vi "Signal Constructor.vi"(8 "error in (no error)":errorcluster, 11 "Signal Settings":T1) -> (0 "error out":errorcluster, 3 "IO Class.lvclass":refnum<class "Signal.lvclass">)   [LabVIEW 2015, in "Signal.lvclass"]
uses:
  Signal.lvclass
  Signal Settings.ctl
  Configuration.ctl
  Digital Indicator/Digital Indicator.lvclass
  Digital Control/Digital Control.lvclass
  Analog Indicator/Analog Indicator.lvclass
  Analog Control/Analog Control.lvclass
  FPGA Addon Input/FPGA Addon Input.lvclass
  FPGA Addon Output/FPGA Addon Output.lvclass
  Wheel Speed Sensor/Wheel Speed Sensor.lvclass
  Signal.lvclass/Signal.ctl
  EST Digital Event/Digital Event.lvclass
  EST Output/EST Output.lvclass
  EST Knock Sensor/Knock Sensor.lvclass
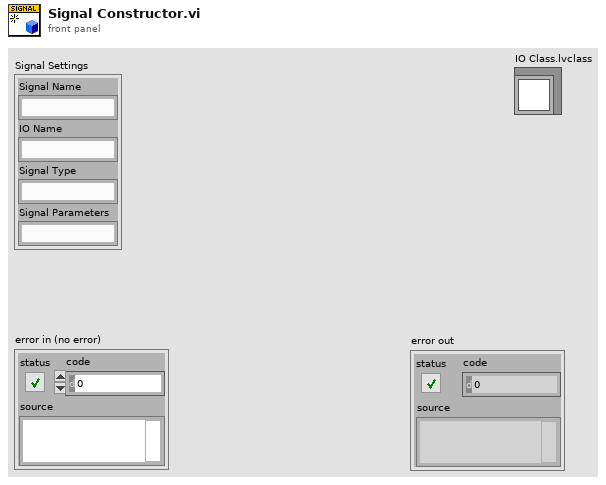
[diagram p1: front panel]
types:
  T1 = typedef "Signal.lvclass/Signal Settings.ctl" = cluster{"Signal Name":string, "IO Name":string, "Signal Type":string, "Signal Parameters":string}
  T2 = typedef "Signal.lvclass/Configuration.ctl" = cluster{"Classification":string, "Direction":string, "Type":string}
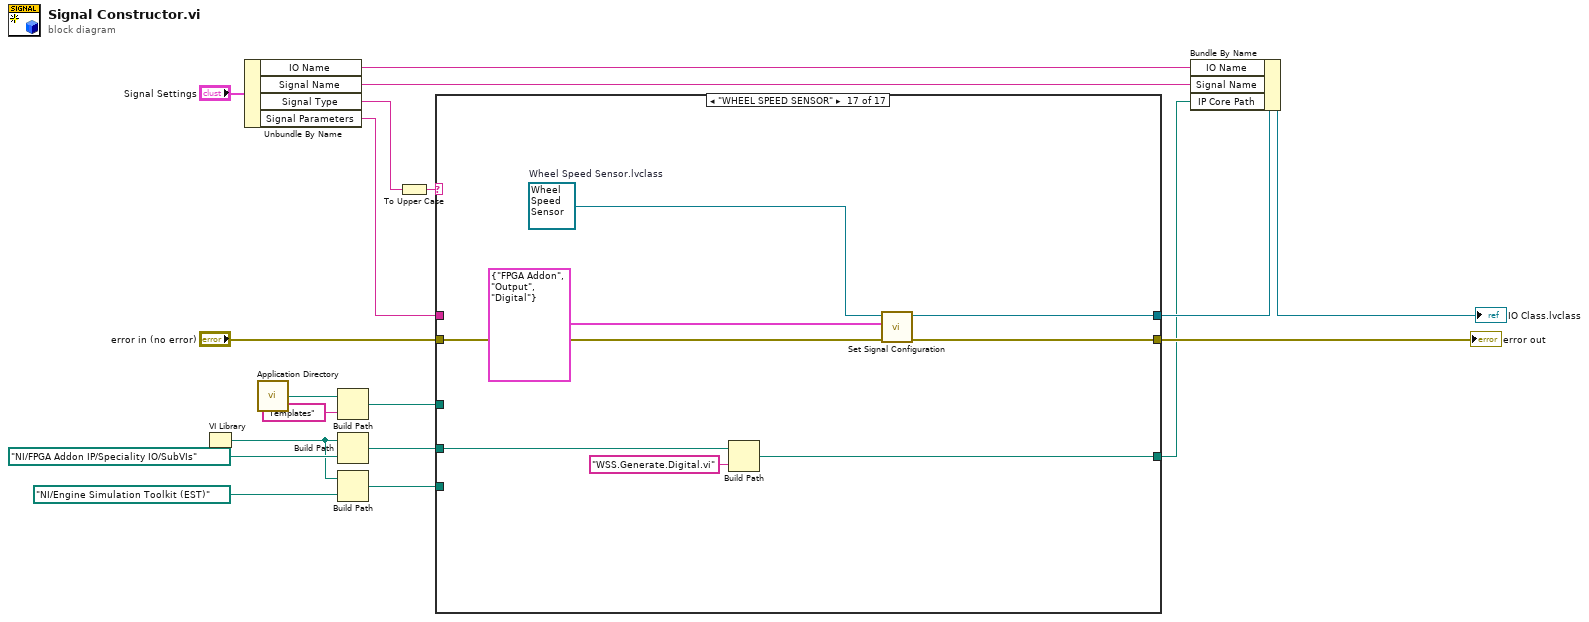
[diagram p0: block diagram]
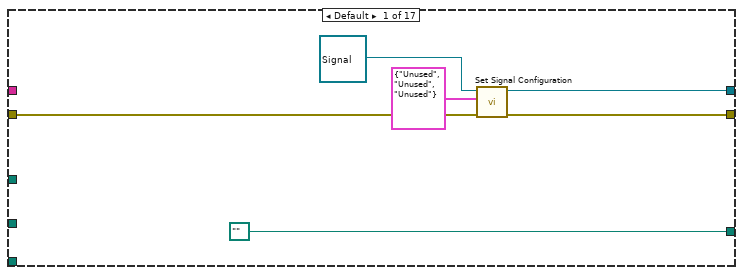
[diagram p2: hidden frame]
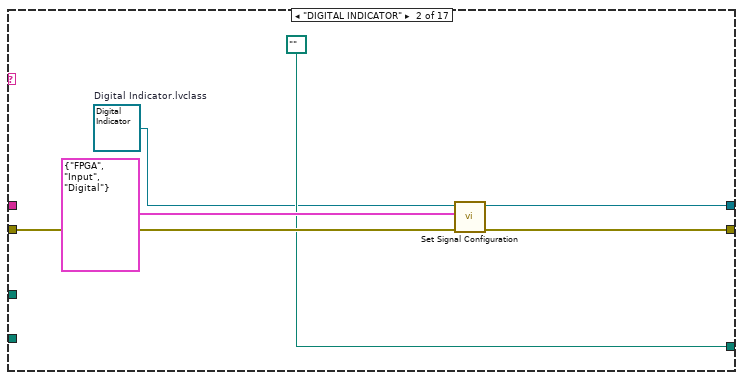
[diagram p3: hidden frame]
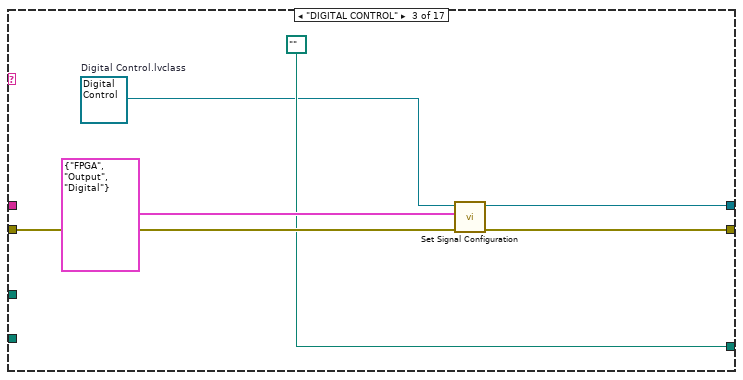
[diagram p4: hidden frame]
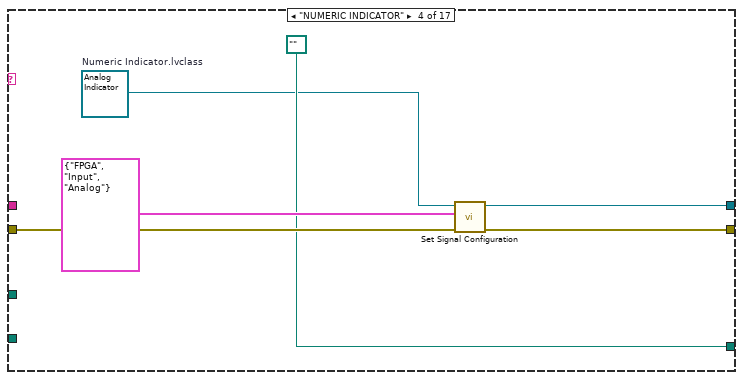
[diagram p5: hidden frame]
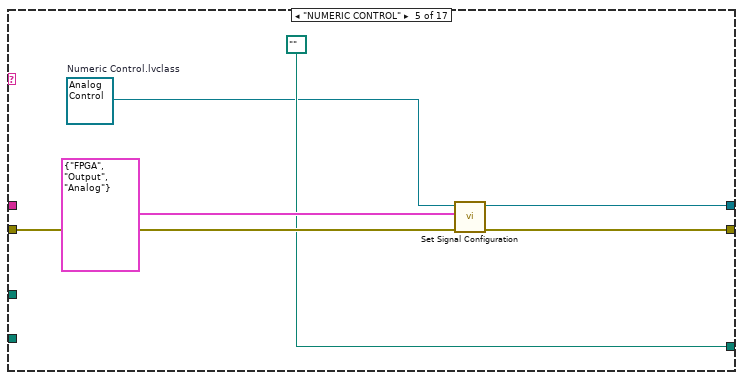
[diagram p6: hidden frame]
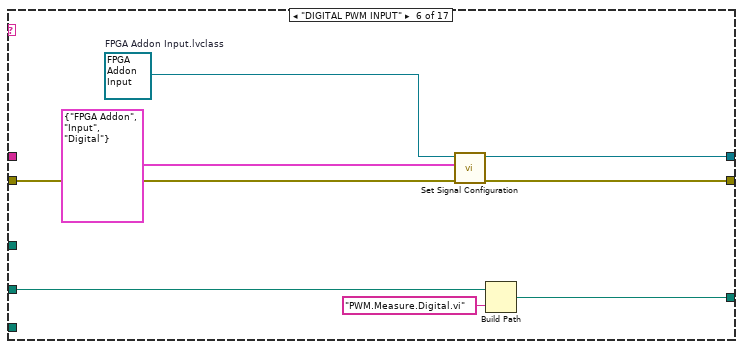
[diagram p7: hidden frame]
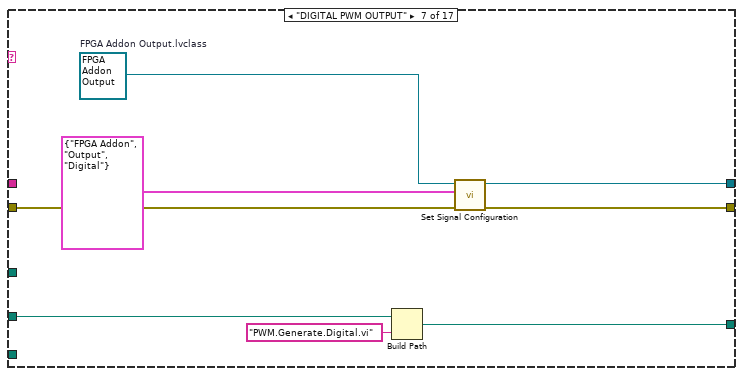
[diagram p8: hidden frame]
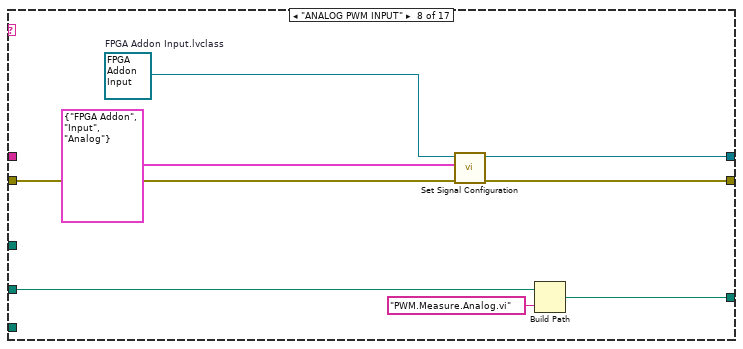
[diagram p9: hidden frame]
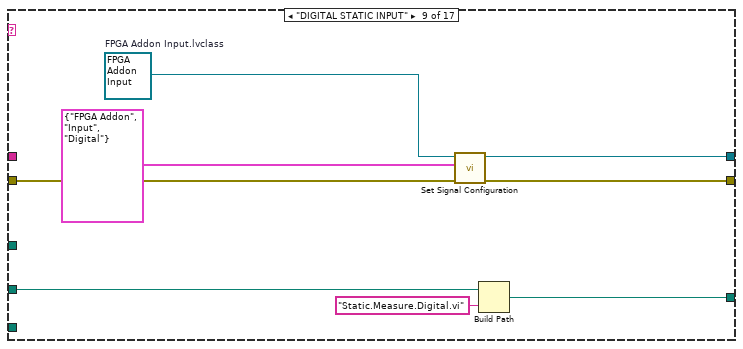
[diagram p10: hidden frame]
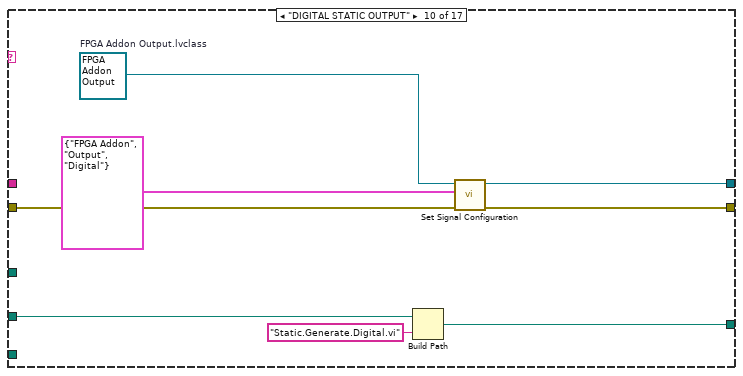
[diagram p11: hidden frame]
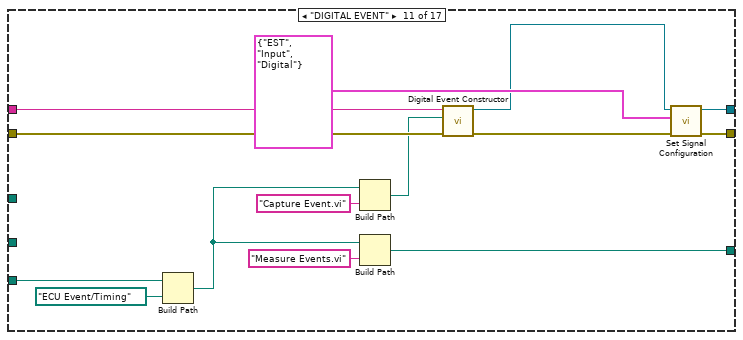
[diagram p12: hidden frame]
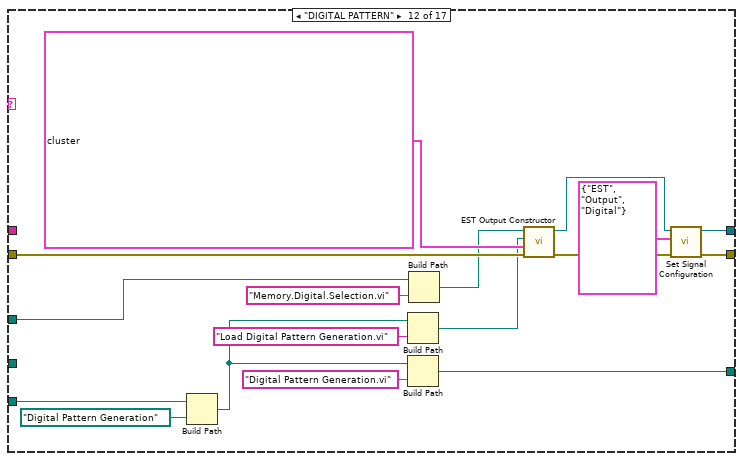
[diagram p13: hidden frame]
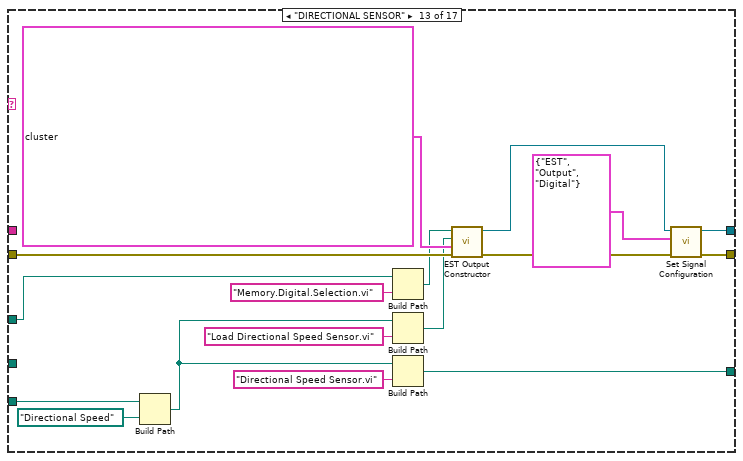
[diagram p14: hidden frame]
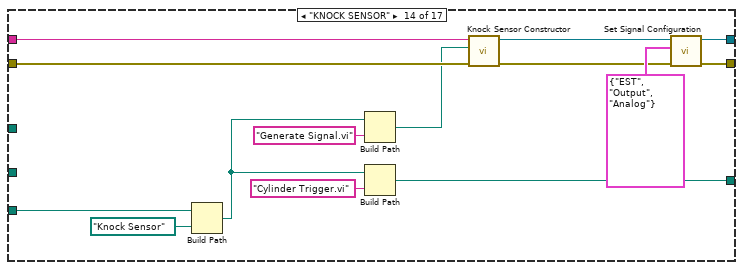
[diagram p15: hidden frame]
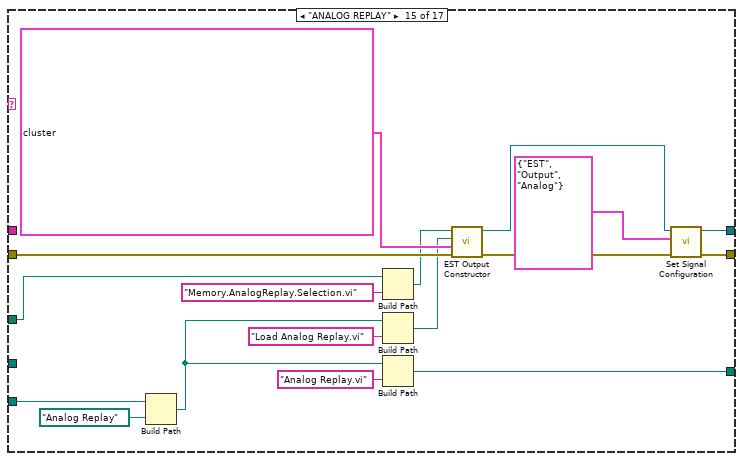
[diagram p16: hidden frame]
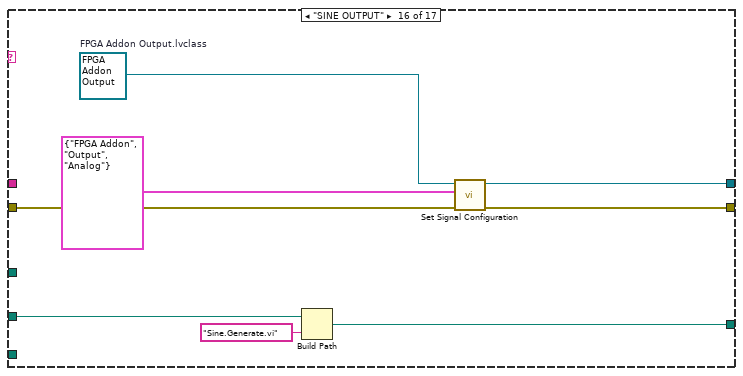
[diagram p17: hidden frame]
diagram:
  n1 = VI Library() -> (path=w6:path)
  n2 = Unbundle By Name("Signal Settings") -> ("IO Name"=w13:string, "Signal Name"=w12:string, "Signal Type"=w18:string, "Signal Parameters"=w11:string)
  n3 = call <vilib>:"Application Directory.vi"() -> ("Application Directory"=w2:path)
  n4 = Build Path(base path=w2, name or relative path="Templates") -> (appended path=w1:path)
  n5 = Build Path(base path=w6, name or relative path=path "NI/FPGA Addon IP/Speciality IO/SubVIs" ("path")) -> (appended path=w5:path)
  n6 = Build Path(base path=w6, name or relative path=path "NI/Engine Simulation Toolkit (EST)" ("path")) -> (appended path=w4:path)
  n7 = To Upper Case(1:w18) -> (0:w17:string)
  n8 = case shown="\"WHEEL SPEED SENSOR\"" w17 {
    tunnel: "error in (no error)" -> [w24 w31 w37 w43 w49 w56 w65 w72 w80 w89 w99 w117 w134 w148 w165 w176 w184]
    tunnel: [w23 w30 w36 w42 w48 w55 w64 w71 w79 w88 w103 w120 w137 w151 w168 w175 w183] -> w15
    tunnel: [w21 w28 w34 w40 w46 w53 w62 w69 w77 w86 w101 w118 w135 w149 w166 w173 w181] -> w10
    tunnel: w11 -> [_ _ _ _ _ _ _ _ _ _ w100 _ _ w145 _ _ _]
    tunnel: [path "" path "" path "" path "" path "" w50 w58 w67 w74 w82 w93 w108 w121 w141 w152 w169 w178] -> w9
    tunnel: w5 -> [_ _ _ _ _ w51 w59 w66 w75 w83 _ _ _ _ _ w171 w180]
    tunnel: w4 -> [_ _ _ _ _ _ _ _ _ _ w96 w109 w124 w142 w156 _ _]
    tunnel: w1 -> [_ _ _ _ _ _ _ _ _ _ _ w106 w129 _ w155 _ _]
    frame Default {
      n9 = call "Set Signal Configuration.vi"("error in (no error)"=w24, "Configuration"=T2 {"Classification"="Unused", "Direction"="Unused", "Type"="Unused"}, "IO Class in"=refnum<class "Signal.lvclass"> refnum ("IO Class.lvclass")) -> ("error out"=w23:errorcluster, "IO Class out"=w21:refnum<class "Signal.lvclass">)  [unwired: 7 in]
    }
    frame "DIGITAL INDICATOR" {
      w26 = refnum<class "Digital Indicator.lvclass"> refnum  # Digital Indicator.lvclass
      n10 = call "Set Signal Configuration.vi"("error in (no error)"=w31, "Configuration"=T2 {"Classification"="FPGA", "Direction"="Input", "Type"="Digital"}, "IO Class in"=w26) -> ("error out"=w30:errorcluster, "IO Class out"=w28:refnum<class "Digital Indicator.lvclass">)  [unwired: 7 in]
    }
    frame "DIGITAL CONTROL" {
      w32 = refnum<class "Digital Control.lvclass"> refnum  # Digital Control.lvclass
      n11 = call "Set Signal Configuration.vi"("error in (no error)"=w37, "Configuration"=T2 {"Classification"="FPGA", "Direction"="Output", "Type"="Digital"}, "IO Class in"=w32) -> ("error out"=w36:errorcluster, "IO Class out"=w34:refnum<class "Digital Control.lvclass">)  [unwired: 7 in]
    }
    frame "NUMERIC INDICATOR" {
      w38 = refnum<class "Analog Indicator.lvclass"> refnum  # Numeric Indicator.lvclass
      n12 = call "Set Signal Configuration.vi"("error in (no error)"=w43, "Configuration"=T2 {"Classification"="FPGA", "Direction"="Input", "Type"="Analog"}, "IO Class in"=w38) -> ("error out"=w42:errorcluster, "IO Class out"=w40:refnum<class "Analog Indicator.lvclass">)  [unwired: 7 in]
    }
    frame "NUMERIC CONTROL" {
      w44 = refnum<class "Analog Control.lvclass"> refnum  # Numeric Control.lvclass
      n13 = call "Set Signal Configuration.vi"("error in (no error)"=w49, "Configuration"=T2 {"Classification"="FPGA", "Direction"="Output", "Type"="Analog"}, "IO Class in"=w44) -> ("error out"=w48:errorcluster, "IO Class out"=w46:refnum<class "Analog Control.lvclass">)  [unwired: 7 in]
    }
    frame "DIGITAL PWM INPUT" {
      w57 = refnum<class "FPGA Addon Input.lvclass"> refnum  # FPGA Addon Input.lvclass
      n14 = call "Set Signal Configuration.vi"("error in (no error)"=w56, "Configuration"=T2 {"Classification"="FPGA Addon", "Direction"="Input", "Type"="Digital"}, "IO Class in"=w57) -> ("error out"=w55:errorcluster, "IO Class out"=w53:refnum<class "FPGA Addon Input.lvclass">)  [unwired: 7 in]
      n15 = Build Path(base path=w51, name or relative path="PWM.Measure.Digital.vi") -> (appended path=w50:path)
    }
    frame "DIGITAL PWM OUTPUT" {
      w61 = refnum<class "FPGA Addon Output.lvclass"> refnum  # FPGA Addon Output.lvclass
      n16 = Build Path(base path=w59, name or relative path="PWM.Generate.Digital.vi") -> (appended path=w58:path)
      n17 = call "Set Signal Configuration.vi"("error in (no error)"=w65, "Configuration"=T2 {"Classification"="FPGA Addon", "Direction"="Output", "Type"="Digital"}, "IO Class in"=w61) -> ("error out"=w64:errorcluster, "IO Class out"=w62:refnum<class "FPGA Addon Output.lvclass">)  [unwired: 7 in]
    }
    frame "ANALOG PWM INPUT" {
      w73 = refnum<class "FPGA Addon Input.lvclass"> refnum  # FPGA Addon Input.lvclass
      n18 = call "Set Signal Configuration.vi"("error in (no error)"=w72, "Configuration"=T2 {"Classification"="FPGA Addon", "Direction"="Input", "Type"="Analog"}, "IO Class in"=w73) -> ("error out"=w71:errorcluster, "IO Class out"=w69:refnum<class "FPGA Addon Input.lvclass">)  [unwired: 7 in]
      n19 = Build Path(base path=w66, name or relative path="PWM.Measure.Analog.vi") -> (appended path=w67:path)
    }
    frame "DIGITAL STATIC INPUT" {
      w81 = refnum<class "FPGA Addon Input.lvclass"> refnum  # FPGA Addon Input.lvclass
      n20 = call "Set Signal Configuration.vi"("error in (no error)"=w80, "Configuration"=T2 {"Classification"="FPGA Addon", "Direction"="Input", "Type"="Digital"}, "IO Class in"=w81) -> ("error out"=w79:errorcluster, "IO Class out"=w77:refnum<class "FPGA Addon Input.lvclass">)  [unwired: 7 in]
      n21 = Build Path(base path=w75, name or relative path="Static.Measure.Digital.vi") -> (appended path=w74:path)
    }
    frame "DIGITAL STATIC OUTPUT" {
      w85 = refnum<class "FPGA Addon Output.lvclass"> refnum  # FPGA Addon Output.lvclass
      n22 = Build Path(base path=w83, name or relative path="Static.Generate.Digital.vi") -> (appended path=w82:path)
      n23 = call "Set Signal Configuration.vi"("error in (no error)"=w89, "Configuration"=T2 {"Classification"="FPGA Addon", "Direction"="Output", "Type"="Digital"}, "IO Class in"=w85) -> ("error out"=w88:errorcluster, "IO Class out"=w86:refnum<class "FPGA Addon Output.lvclass">)  [unwired: 7 in]
    }
    frame "DIGITAL EVENT" {
      n24 = Build Path(base path=w96, name or relative path=path "ECU Event/Timing") -> (appended path=w91:path)
      n25 = Build Path(base path=w91, name or relative path="Capture Event.vi") -> (appended path=w90:path)
      n26 = Build Path(base path=w91, name or relative path="Measure Events.vi") -> (appended path=w93:path)
      n27 = call "Digital Event Constructor.vi"("error in (no error)"=w99, "Capture Path"=w90, "Signal Parameters"=w100) -> ("error out"=w98:errorcluster, "Digital Event.lvclass"=w97:refnum<class "Digital Event.lvclass">)  [unwired: 7 in]
      n28 = call "Set Signal Configuration.vi"("error in (no error)"=w98, "Configuration"=T2 {"Classification"="EST", "Direction"="Input", "Type"="Digital"}, "IO Class in"=w97) -> ("error out"=w103:errorcluster, "IO Class out"=w101:refnum<class "Digital Event.lvclass">)  [unwired: 7 in]
    }
    frame "DIGITAL PATTERN" {
      n29 = Build Path(base path=w109, name or relative path=path "Digital Pattern Generation") -> (appended path=w110:path)
      n30 = Build Path(base path=w110, name or relative path="Load Digital Pattern Generation.vi") -> (appended path=w107:path)
      n31 = Build Path(base path=w110, name or relative path="Digital Pattern Generation.vi") -> (appended path=w108:path)
      n32 = Build Path(base path=w106, name or relative path="Memory.Digital.Selection.vi") -> (appended path=w104:path)
      n33 = call "EST Output Constructor.vi"("error in (no error)"=w117, "Project Item"=cluster{"Name":string, "Value":variant}[] [{"Name"="FPGA.PersistentID", "Value"=variant(string "{CD7EB185-1A87-4E78-8C08-5D9A1491F439}")}, {"Name"="fullEmulation", "Value"=variant(bool TRUE)}, {"Name"="Memory Latency", "Value"=variant(u32 1)}, {"Name"="Multiple Clock Domains", "Value"=variant(bool FALSE)}, {"Name"="NI.LV.FPGA.CompileConfigString", "Value"=variant(string "Actual Number of Elements=1024;ReadArbs=2;WriteArbs=2;Implementation=2;DataType=100080000000000100094006000355313600010000000000000000;InitDataHash=;DRAM Selection=DramBank0;DRAM Max Outstanding Requests=64;DRAM Include Byte Enables=FALSE;DRAM Grant Time=50;Interface Configuration=Read A-Write B;Multiple Clock Domains=FALSE;Memory Latency=1")}, {"Name"="NI.LV.FPGA.MEMORY.ActualNumberOfElements", "Value"=variant(u32 1024)}, {"Name"="NI.LV.FPGA.MEMORY.DataWidth", "Value"=variant(u32 6)}, {"Name"="NI.LV.FPGA.MEMORY.DramIncludeByteEnables", "Value"=variant(bool FALSE)}, {"Name"="NI.LV.FPGA.MEMORY.DramMaxOutstandingRequests", "Value"=variant(i32 64)}, {"Name"="NI.LV.FPGA.MEMORY.DramSelection", "Value"=variant(string "DramBank0")}, {"Name"="NI.LV.FPGA.MEMORY.Init", "Value"=variant(bool FALSE)}, {"Name"="NI.LV.FPGA.MEMORY.InitData", "Value"=variant(string "")}, {"Name"="NI.LV.FPGA.MEMORY.InitVIPath", "Value"=variant(string "")}, {"Name"="NI.LV.FPGA.MEMORY.InterfaceAArbitration", "Value"=variant(u32 2)}, {"Name"="NI.LV.FPGA.MEMORY.InterfaceBArbitration", "Value"=variant(u32 2)}, {"Name"="NI.LV.FPGA.MEMORY.InterfaceConfig", "Value"=variant(u32 0)}, {"Name"="NI.LV.FPGA.MEMORY.RequestedNumberOfElements", "Value"=variant(u32 1024)}, {"Name"="NI.LV.FPGA.MEMORY.Type", "Value"=variant(u32 2)}, {"Name"="NI.LV.FPGA.ScriptConfigString", "Value"=variant(string "Actual Number of Elements=1024;ReadArbs=2;WriteArbs=2;Implementation=2;DataType=100080000000000100094006000355313600010000000000000000;InitDataHash=;DRAM Selection=DramBank0;DRAM Max Outstanding Requests=64;DRAM Include Byte Enables=FALSE;DRAM Grant Time=50;Interface Configuration=Read A-Write B;Multiple Clock Domains=FALSE;Memory Latency=1Persist Memory ValuesTRUE;")}, {"Name"="NI.LV.FPGA.Valid", "Value"=variant(bool TRUE)}, {"Name"="NI.LV.FPGA.Version", "Value"=variant(i32 10)}, {"Name"="Type Descriptor", "Value"=variant(string "100080000000000100094006000355313600010000000000000000")}] ("Array 2"), "Load Path"=w107, "Memory Template Path"=w104) -> ("error out"=w116:errorcluster, "EST Output.lvclass"=w115:refnum<class "EST Output.lvclass">)  [unwired: 6 in]
      n34 = call "Set Signal Configuration.vi"("error in (no error)"=w116, "Configuration"=T2 {"Classification"="EST", "Direction"="Output", "Type"="Digital"}, "IO Class in"=w115) -> ("error out"=w120:errorcluster, "IO Class out"=w118:refnum<class "EST Output.lvclass">)  [unwired: 7 in]
    }
    frame "DIRECTIONAL SENSOR" {
      n35 = Build Path(base path=w124, name or relative path=path "Directional Speed") -> (appended path=w123:path)
      n36 = Build Path(base path=w129, name or relative path="Memory.Digital.Selection.vi") -> (appended path=w128:path)
      n37 = Build Path(base path=w123, name or relative path="Load Directional Speed Sensor.vi") -> (appended path=w122:path)
      n38 = Build Path(base path=w123, name or relative path="Directional Speed Sensor.vi") -> (appended path=w121:path)
      n39 = call "EST Output Constructor.vi"("error in (no error)"=w134, "Project Item"=cluster{"Name":string, "Value":variant}[] [{"Name"="FPGA.PersistentID", "Value"=variant(string "{CD7EB185-1A87-4E78-8C08-5D9A1491F439}")}, {"Name"="fullEmulation", "Value"=variant(bool TRUE)}, {"Name"="Memory Latency", "Value"=variant(u32 1)}, {"Name"="Multiple Clock Domains", "Value"=variant(bool FALSE)}, {"Name"="NI.LV.FPGA.CompileConfigString", "Value"=variant(string "Actual Number of Elements=1024;ReadArbs=2;WriteArbs=2;Implementation=2;DataType=100080000000000100094006000355313600010000000000000000;InitDataHash=;DRAM Selection=DramBank0;DRAM Max Outstanding Requests=64;DRAM Include Byte Enables=FALSE;DRAM Grant Time=50;Interface Configuration=Read A-Write B;Multiple Clock Domains=FALSE;Memory Latency=1")}, {"Name"="NI.LV.FPGA.MEMORY.ActualNumberOfElements", "Value"=variant(u32 1024)}, {"Name"="NI.LV.FPGA.MEMORY.DataWidth", "Value"=variant(u32 6)}, {"Name"="NI.LV.FPGA.MEMORY.DramIncludeByteEnables", "Value"=variant(bool FALSE)}, {"Name"="NI.LV.FPGA.MEMORY.DramMaxOutstandingRequests", "Value"=variant(i32 64)}, {"Name"="NI.LV.FPGA.MEMORY.DramSelection", "Value"=variant(string "DramBank0")}, {"Name"="NI.LV.FPGA.MEMORY.Init", "Value"=variant(bool FALSE)}, {"Name"="NI.LV.FPGA.MEMORY.InitData", "Value"=variant(string "")}, {"Name"="NI.LV.FPGA.MEMORY.InitVIPath", "Value"=variant(string "")}, {"Name"="NI.LV.FPGA.MEMORY.InterfaceAArbitration", "Value"=variant(u32 2)}, {"Name"="NI.LV.FPGA.MEMORY.InterfaceBArbitration", "Value"=variant(u32 2)}, {"Name"="NI.LV.FPGA.MEMORY.InterfaceConfig", "Value"=variant(u32 0)}, {"Name"="NI.LV.FPGA.MEMORY.RequestedNumberOfElements", "Value"=variant(u32 1024)}, {"Name"="NI.LV.FPGA.MEMORY.Type", "Value"=variant(u32 2)}, {"Name"="NI.LV.FPGA.ScriptConfigString", "Value"=variant(string "Actual Number of Elements=1024;ReadArbs=2;WriteArbs=2;Implementation=2;DataType=100080000000000100094006000355313600010000000000000000;InitDataHash=;DRAM Selection=DramBank0;DRAM Max Outstanding Requests=64;DRAM Include Byte Enables=FALSE;DRAM Grant Time=50;Interface Configuration=Read A-Write B;Multiple Clock Domains=FALSE;Memory Latency=1Persist Memory ValuesTRUE;")}, {"Name"="NI.LV.FPGA.Valid", "Value"=variant(bool TRUE)}, {"Name"="NI.LV.FPGA.Version", "Value"=variant(i32 10)}, {"Name"="Type Descriptor", "Value"=variant(string "100080000000000100094006000355313600010000000000000000")}] ("Array 2"), "Load Path"=w122, "Memory Template Path"=w128) -> ("error out"=w133:errorcluster, "EST Output.lvclass"=w132:refnum<class "EST Output.lvclass">)  [unwired: 6 in]
      n40 = call "Set Signal Configuration.vi"("error in (no error)"=w133, "Configuration"=T2 {"Classification"="EST", "Direction"="Output", "Type"="Digital"}, "IO Class in"=w132) -> ("error out"=w137:errorcluster, "IO Class out"=w135:refnum<class "EST Output.lvclass">)  [unwired: 7 in]
    }
    frame "KNOCK SENSOR" {
      n41 = Build Path(base path=w142, name or relative path=path "Knock Sensor") -> (appended path=w139:path)
      n42 = Build Path(base path=w139, name or relative path="Generate Signal.vi") -> (appended path=w138:path)
      n43 = Build Path(base path=w139, name or relative path="Cylinder Trigger.vi") -> (appended path=w141:path)
      n44 = call "Knock Sensor Constructor.vi"("error in (no error)"=w148, "Generate Signal Path"=w138, "Signal Parameters"=w145) -> ("error out"=w147:errorcluster, "EST Knock Sensor.lvclass"=w146:refnum<class "Knock Sensor.lvclass">)  [unwired: 7 in]
      n45 = call "Set Signal Configuration.vi"("error in (no error)"=w147, "Configuration"=T2 {"Classification"="EST", "Direction"="Output", "Type"="Analog"}, "IO Class in"=w146) -> ("error out"=w151:errorcluster, "IO Class out"=w149:refnum<class "Knock Sensor.lvclass">)  [unwired: 7 in]
    }
    frame "ANALOG REPLAY" {
      n46 = Build Path(base path=w156, name or relative path=path "Analog Replay") -> (appended path=w157:path)
      n47 = Build Path(base path=w155, name or relative path="Memory.AnalogReplay.Selection.vi") -> (appended path=w153:path)
      n48 = Build Path(base path=w157, name or relative path="Load Analog Replay.vi") -> (appended path=w154:path)
      n49 = Build Path(base path=w157, name or relative path="Analog Replay.vi") -> (appended path=w152:path)
      n50 = call "EST Output Constructor.vi"("error in (no error)"=w165, "Project Item"=cluster{"Name":string, "Value":variant}[] [{"Name"="FPGA.PersistentID", "Value"=variant(string "{CD7EB185-1A87-4E78-8C08-5D9A1491F439}")}, {"Name"="fullEmulation", "Value"=variant(bool TRUE)}, {"Name"="Memory Latency", "Value"=variant(u32 1)}, {"Name"="Multiple Clock Domains", "Value"=variant(bool FALSE)}, {"Name"="NI.LV.FPGA.CompileConfigString", "Value"=variant(string "Actual Number of Elements=16384;ReadArbs=2;WriteArbs=2;Implementation=2;DataType=100080000000000100094002000349313600010000000000000000;InitDataHash=;DRAM Selection=DramBank0;DRAM Max Outstanding Requests=64;DRAM Include Byte Enables=FALSE;DRAM Grant Time=50;Interface Configuration=Read A-Write B;Multiple Clock Domains=FALSE;Memory Latency=1")}, {"Name"="NI.LV.FPGA.MEMORY.ActualNumberOfElements", "Value"=variant(u32 16384)}, {"Name"="NI.LV.FPGA.MEMORY.DataWidth", "Value"=variant(u32 2)}, {"Name"="NI.LV.FPGA.MEMORY.DramIncludeByteEnables", "Value"=variant(bool FALSE)}, {"Name"="NI.LV.FPGA.MEMORY.DramMaxOutstandingRequests", "Value"=variant(i32 64)}, {"Name"="NI.LV.FPGA.MEMORY.DramSelection", "Value"=variant(string "DramBank0")}, {"Name"="NI.LV.FPGA.MEMORY.Init", "Value"=variant(bool FALSE)}, {"Name"="NI.LV.FPGA.MEMORY.InitData", "Value"=variant(string "")}, {"Name"="NI.LV.FPGA.MEMORY.InitVIPath", "Value"=variant(string "")}, {"Name"="NI.LV.FPGA.MEMORY.InterfaceAArbitration", "Value"=variant(u32 2)}, {"Name"="NI.LV.FPGA.MEMORY.InterfaceBArbitration", "Value"=variant(u32 2)}, {"Name"="NI.LV.FPGA.MEMORY.InterfaceConfig", "Value"=variant(u32 0)}, {"Name"="NI.LV.FPGA.MEMORY.RequestedNumberOfElements", "Value"=variant(u32 16384)}, {"Name"="NI.LV.FPGA.MEMORY.Type", "Value"=variant(u32 2)}, {"Name"="NI.LV.FPGA.ScriptConfigString", "Value"=variant(string "Actual Number of Elements=16384;ReadArbs=2;WriteArbs=2;Implementation=2;DataType=100080000000000100094002000349313600010000000000000000;InitDataHash=;DRAM Selection=DramBank0;DRAM Max Outstanding Requests=64;DRAM Include Byte Enables=FALSE;DRAM Grant Time=50;Interface Configuration=Read A-Write B;Multiple Clock Domains=FALSE;Memory Latency=1Persist Memory ValuesTRUE;")}, {"Name"="NI.LV.FPGA.Valid", "Value"=variant(bool TRUE)}, {"Name"="NI.LV.FPGA.Version", "Value"=variant(i32 10)}, {"Name"="Type Descriptor", "Value"=variant(string "100080000000000100094002000349313600010000000000000000")}] ("Array 2"), "Load Path"=w154, "Memory Template Path"=w153) -> ("error out"=w164:errorcluster, "EST Output.lvclass"=w163:refnum<class "EST Output.lvclass">)  [unwired: 6 in]
      n51 = call "Set Signal Configuration.vi"("error in (no error)"=w164, "Configuration"=T2 {"Classification"="EST", "Direction"="Output", "Type"="Analog"}, "IO Class in"=w163) -> ("error out"=w168:errorcluster, "IO Class out"=w166:refnum<class "EST Output.lvclass">)  [unwired: 7 in]
    }
    frame "SINE OUTPUT" {
      w172 = refnum<class "FPGA Addon Output.lvclass"> refnum  # FPGA Addon Output.lvclass
      n52 = Build Path(base path=w171, name or relative path="Sine.Generate.vi") -> (appended path=w169:path)
      n53 = call "Set Signal Configuration.vi"("error in (no error)"=w176, "Configuration"=T2 {"Classification"="FPGA Addon", "Direction"="Output", "Type"="Analog"}, "IO Class in"=w172) -> ("error out"=w175:errorcluster, "IO Class out"=w173:refnum<class "FPGA Addon Output.lvclass">)  [unwired: 7 in]
    }
    frame "WHEEL SPEED SENSOR" {
      w177 = refnum<class "Wheel Speed Sensor.lvclass"> refnum  # Wheel Speed Sensor.lvclass
      n54 = Build Path(base path=w180, name or relative path="WSS.Generate.Digital.vi") -> (appended path=w178:path)
      n55 = call "Set Signal Configuration.vi"("error in (no error)"=w184, "Configuration"=T2 {"Classification"="FPGA Addon", "Direction"="Output", "Type"="Digital"}, "IO Class in"=w177) -> ("error out"=w183:errorcluster, "IO Class out"=w181:refnum<class "Wheel Speed Sensor.lvclass">)  [unwired: 7 in]
    }
  }
  "error out" <- w15
  n56 = Bundle By Name(cluster=w10, "IO Name"=w13, "Signal Name"=w12, "IP Core Path"=w9) -> (→"IO Class.lvclass":refnum<class "Signal.lvclass">)
